vi "Send VHM-continiousDataSet.vi"(7 "Message Priority (Normal)":T2=enum."Normal", 8 "error in (no error)":errorcluster, 10 "Read Option":T1, 11 "Message Enqueuer":refnum<class "Message Enqueuer.lvclass">) -> (0 "error out":errorcluster, 3 "Message Enqueuer out":refnum<class "Message Enqueuer.lvclass">)   [LabVIEW 2020, in "VHM-VNA_Hardware_Manager.lvlib" / "VHM-continiousDataSet Msg.lvclass"]
doc: "This VI sends the message to an actor."
uses:
  VHM-continiousDataSet Msg.lvclass
  <vilib>/ActorFramework/Message Enqueuer/Message Enqueuer.lvclass
  <vilib>/ActorFramework/Message Enqueuer/Message Priority.ctl
  VHM-VNA_Hardware_Manager/VHM-continuous_get_clust.ctl
  C:/Program Files (x86)/National Instruments/LabVIEW 2020/vi.lib/ActorFramework/Message/Message.lvclass
  VHM-continiousDataSet Msg.lvclass/VHM-continiousDataSet Msg.ctl
  <vilib>/ActorFramework/Message Enqueuer/Message Enqueuer.lvclass/Message Enqueuer.ctl
  <vilib>/ActorFramework/Message Priority Queue/Priority Enqueue.vi
  VHM-VNA_Hardware_Manager/VHM-VNA_Hardware_Manager.lvclass
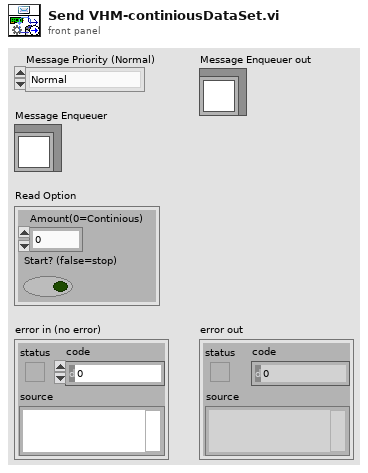
[diagram p1: front panel]
types:
  T1 = typedef "VHM-VNA_Hardware_Manager.lvlib/VHM-VNA_Hardware_Manager.lvclass/VHM-continuous_get_clust.ctl" = cluster{"Amount(0=Continious)":u8, "Start? (false=stop)":bool}
  T2 = typedef "Actor Framework.lvlib/Message Enqueuer.lvclass/Message Priority.ctl" = enum16{"Low", "Normal", "High"}
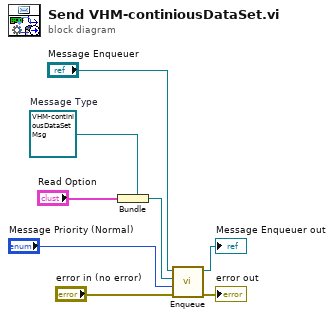
[diagram p0: block diagram]
diagram:
  w5 = refnum<class "VHM-continiousDataSet Msg.lvclass"> refnum  # Message Type
  n1 = Bundle(cluster=w5, "Read Option") -> (w4:refnum<class "VHM-continiousDataSet Msg.lvclass">)
  n2 = call <vilib>:"Enqueue.vi"("error in (no error)"="error in (no error)", "Message Priority (Normal)"="Message Priority (Normal)", "Message"=w4, "Message Enqueuer in"="Message Enqueuer") -> ("error out"=→"error out":errorcluster, "Message Enqueuer out"=→"Message Enqueuer out":refnum<class "Message Enqueuer.lvclass">)  [unwired: 6 in]
